vi "VeristandInitialize.vi"(10 "Visible":bool) -> (0 "error out":errorcluster)   [LabVIEW 2020, in "ni-veristand-steps-runtime-lib.lvlib"]
uses:
  ni-veristand-steps-runtime-lib.lvlib
  NationalInstruments.VeriStand.ClientAPI
  <vilib>/NI VeriStand/Execution/Project/NI_VS Project ExecutionAPI.lvlib
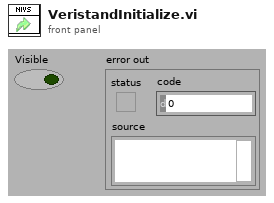
[diagram p1: front panel]
types:
  T1 = typedef "ni-veristand-steps-runtime-lib.lvlib/VeriStand dotNet References.ctl" = cluster{"ModelManager":T2, "AlarmManager":T3, "ChannelFault":T4, "WorkspaceManager":T5, "Project Ref":T6}
  T2 = typedef "NI_VS ModelManager ExecutionAPI.lvlib/ModelManagerAPI.ctl" = refnum<k24>
  T3 = typedef "NI_VS AlarmManager ExecutionAPI.lvlib/AlarmManagerAPI.ctl" = refnum<k24>
  T4 = typedef "NI_VS ChannelFault ExecutionAPI.lvlib/ChannelFaultAPI.ctl" = refnum<k24>
  T5 = typedef "NI_VS Workspace ExecutionAPI.lvlib/WorkspaceAPI.ctl" = refnum<k24>
  T6 = typedef "NI_VS Project ExecutionAPI.lvlib/Project Ref.ctl" = refnum<k24>
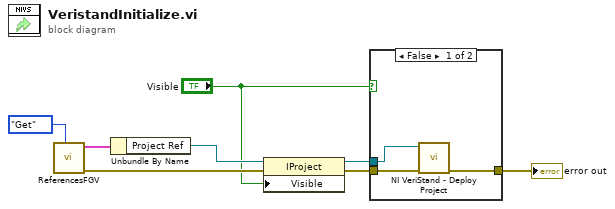
[diagram p0: block diagram]
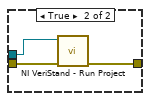
[diagram p2: hidden frame]
diagram:
  n1 = call "ReferencesFGV.vi"("Get/Set"=enum16{"Get", "Set"}."Get") -> ("error out"=w5:errorcluster, "VeriStand dotNET Refs out"=w7:T1)  [unwired: 9 in]
  n2 = Unbundle By Name(w7) -> ("Project Ref"=w6:T6)
  n3 = property class="IProject"(reference=w6, error in=w5, "Visible"="Visible") -> (reference out=w2:T6, error out=w3:errorcluster)
  n4 = case shown="False" "Visible" {
    tunnel: w3 -> [w11 w14]
    tunnel: w2 -> [w9 w12]
    tunnel: [w10 w13] -> w1
    frame False {
      n5 = call <vilib>:"NI VeriStand - Deploy Project.vi"("error in (no error)"=w11, "Project Ref in"=w9) -> ("error out"=w10:errorcluster)  [unwired: 8 in, 1 out]
    }
    frame True {
      n6 = call <vilib>:"NI VeriStand - Run Project.vi"("error in (no error)"=w14, "Project Ref in"=w12) -> ("error out"=w13:errorcluster)  [unwired: 8 in, 1 out]
    }
  }
  "error out" <- w1
